vi "INI Input Clusters.vi"() -> (0 "File output directories":T2={"Archive Location"=path "", "Archive Location 2"=path "<Not A Path>", "OutPut Path"=path "", "Directory(s) To Scan Files"=[]}, 1 "FTP CRED Cluster":T4={"Host"="", "UserName"="", "PassWord"="", "FTP File Path"="", "FTP Timeout (S)"=60, "Active or Passive"=FALSE, "ASCII or Binary"=FALSE} {"FTP Timeout (S)" min=0 max=300 step=1}, 2 "Email Notification Cluster":T3, 3 "Email Recipiant List":string[](array[string]), 4 "error out":errorcluster, 5 "time stamp":timestamp, 6 "Site ID":string, 7 "File Management cluster":T1, 8 "Auto FTP":bool, 9 "Auto Archive":bool, 11 "hours old date mod(hours)":u8=2)   [LabVIEW 2011]
uses:
  Controls/FTP Credintials.ctl
  Controls/Ping address and email notify.ctl
  Controls/File Path directories.ctl
  Controls/File Management.ctl
  <vilib>/Utility/sysdir.llb/System Directory Type.ctl
  <vilib>/Utility/config.llb/Read Key (String).vi
  <vilib>/Utility/config.llb/Read Key (Boolean).vi
  <vilib>/Utility/config.llb/Read Key (Path).vi
  <vilib>/Utility/config.llb/Read Key (I32).vi
  <vilib>/Utility/config.llb/Read Key (U32).vi
  <vilib>/Utility/config.llb/NI_LVConfig.lvlib
panel:
  # "File Handling Method"
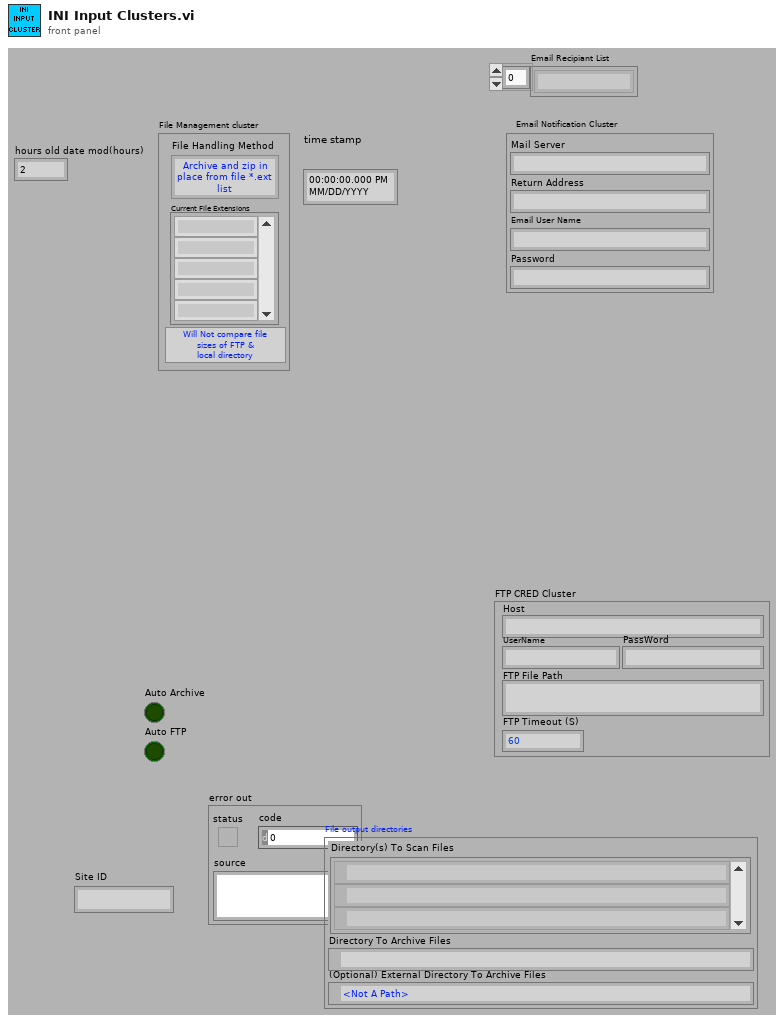
[diagram p1: front panel]
types:
  T1 = typedef "File Management.ctl" = cluster{"Comp File Size":bool, "File Handle Method":enum16{"Archive and zip in place from file *.ext list", "Archive and zip ALL file Types to archive directory", "Archive and zip to archive directory from file *.ext list", "Perform no file management"}, "file extention list":string[]}
  T2 = typedef "File Path directories.ctl" = cluster{"Archive Location":path, "Archive Location 2":path, "OutPut Path":path, "Directory(s) To Scan Files":path[]}
  T3 = typedef "Ping address and email notify.ctl" = cluster{"Mail Server":string, "Return Address":string, "Email User Name":string, "Password":string}
  T4 = typedef "FTP Credintials.ctl" = cluster{"Host":string, "UserName":string, "PassWord":string, "FTP File Path":string, "FTP Timeout (S)":i32, "Active or Passive":bool, "ASCII or Binary":bool}
  T5 = enum16{"Archive and Zip IN Place", "Archive and Zip All File Types", "Archive and Zip from List of File Extensions ", "Perform No File Management"}
  T6 = typedef "System Directory Type.ctl" = i32
  T7 = typedef "NI_LVConfig.lvlib/Config Data RefNum.ctl" = refnum<k1>
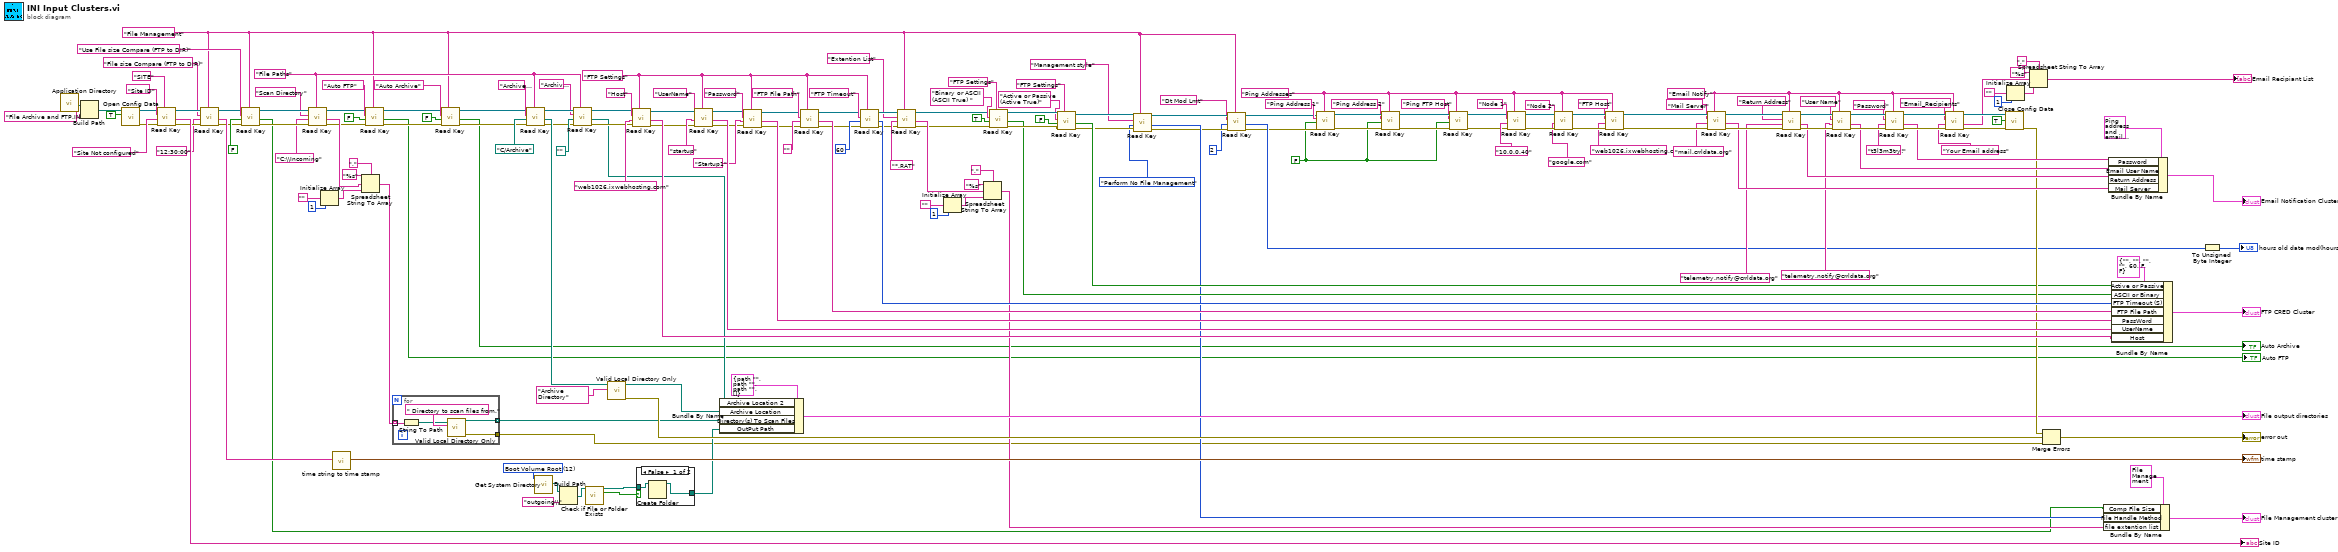
[diagram p0: block diagram]
diagram:
  w1 = FALSE
  w27 = "File Management" ("section")
  w77 = T6 12 items=["User Home"=0, "User Desktop"=1, "User Documents"=2, "User Application Data"=3, "User Preferences"=4, "User Temporary"=5, "Public Documents"=6, "Public Application Data"=7, "Public Preferences"=8, "Public Cache"=13, "System Core Libraries"=9, "System Installed Libraries"=10, "Application Files"=11, "Boot Volume Root"=12] ("system directory type")
  w102 = "FTP Settings" ("name or relative path")
  w91 = "File Paths" ("name or relative path")
  w2 = "Ping Addresses" ("name or relative path")
  w192 = "Email Notify" ("name or relative path")
  n1 = call <vilib>:"Application Directory.vi"() -> ("Application Directory"=w16:path)
  n2 = Build Path(base path=w16, name or relative path="File Archive and FTP.INI") -> (appended path=w140:path)
  n3 = call <vilib>:"Open Config Data.vi"("create file if necessary (T)"=TRUE, "configuration file path"=w140) -> ("error out"=w129:errorcluster, "refnum"=w130:T7)  [unwired: 7 in, 1 out]
  n4 = call-poly <vilib>:"Read Key.vi"("section"="SITE" ("name or relative path"), "error in (no error)"=w129, "default value"="Site Not configured", "key"="Site ID" ("name or relative path"), "refnum"=w130) -> ("error out"=w132:errorcluster, "value"=→"Site ID":string, "refnum out"=w131:T7)  [unwired: 3 in, 1 out]
  n5 = call-poly <vilib>:"Read Key.vi"("section"=w27, "error in (no error)"=w132, "default value"="12:30:00", "key"="File size Compare (FTP to DIR)" ("name or relative path"), "refnum"=w131) -> ("error out"=w120:errorcluster, "value"=w127:string, "refnum out"=w121:T7)  [unwired: 3 in, 1 out]
  n6 = call-poly <vilib>:"Read Key.vi"("section"=w27, "error in (no error)"=w120, "default value"=FALSE ("create file if necessary (T)"), "key"="Use File size Compare (FTP to DIR)" ("name or relative path"), "refnum"=w121) -> ("error out"=w123:errorcluster, "value"=w50:bool, "refnum out"=w122:T7)  [unwired: 3 in, 1 out]
  n7 = call-poly <vilib>:"Read Key.vi"("section"=w91, "error in (no error)"=w123, "default value"="C:\\Incoming", "key"="Scan Directory" ("name or relative path"), "refnum"=w122) -> ("error out"=w23:errorcluster, "value"=w39:string, "refnum out"=w26:T7)  [unwired: 3 in, 1 out]
  n8 = Initialize Array("", 1 ("dimension size")) -> (w40:string[])
  n9 = call "time string to time stamp.vi"("time string example(16:15:00)"=w127) -> ("time stamp"=→"time stamp":timestamp)  [unwired: 10 in]
  n10 = Spreadsheet String To Array(delimiter (Tab)=",", format string="%s", spreadsheet string=w39, array type (2D Dbl)=w40) -> (array=w38:string[])
  n11 = call-poly <vilib>:"Read Key.vi"("section"=w27, "error in (no error)"=w23, "default value"=FALSE, "key"="Auto FTP" ("name or relative path"), "refnum"=w26) -> ("error out"=w22:errorcluster, "value"=→"Auto FTP":bool, "refnum out"=w25:T7)  [unwired: 3 in, 1 out]
  n12 = for {
    tunnel: w38 -> [w199] mode=indexing
    tunnel: [w196] -> w37 mode=indexing
    tunnel: [w195] -> w36
    n13 = String To Path(string=w199) -> (path=w197:path)
    n14 = call "Valid Local Directory Only.vi"("Directory ref"=" Directory to scan files from.", "Path input"=w197) -> ("error out"=w195:errorcluster, "Path output"=w196:path)  [unwired: 8 in]
  }
  n15 = call-poly <vilib>:"Read Key.vi"("section"=w27, "error in (no error)"=w22, "default value"=FALSE, "key"="Auto Archive" ("name or relative path"), "refnum"=w25) -> ("error out"=w21:errorcluster, "value"=→"Auto Archive":bool, "refnum out"=w24:T7)  [unwired: 3 in, 1 out]
  n16 = call-poly <vilib>:"Read Key.vi"("section"=w91, "error in (no error)"=w21, "default value"=path "C:/Archive", "key"="Archive location 1" ("name or relative path"), "refnum"=w24) -> ("error out"=w89:errorcluster, "value"=w138:path, "refnum out"=w88:T7)  [unwired: 3 in, 1 out]
  n17 = call <vilib>:"Get System Directory.vi"("system directory type"=w77) -> ("system directory"=w76:path)  [unwired: 10 in]
  n18 = Build Path(base path=w76, name or relative path="outgoing\\") -> (appended path=w79:path)
  n19 = call-poly <vilib>:"Read Key.vi"("section"=w91, "error in (no error)"=w89, "default value"=path "", "key"="Archive location 2" ("name or relative path"), "refnum"=w88) -> ("error out"=w92:errorcluster, "value"=w85:path, "refnum out"=w97:T7)  [unwired: 3 in, 1 out]
  n20 = call <vilib>:"Check if File or Folder Exists.vi"("path"=w79) -> ("file or folder exists?"=w75:bool, "dup path"=w74:path)  [unwired: 8 in, 1 out]
  n21 = call "Valid Local Directory Only.vi"("Directory ref"="Archive Directory", "Path input"=w138) -> ("error out"=w141:errorcluster, "Path output"=w81:path)  [unwired: 8 in]
  n22 = call-poly <vilib>:"Read Key.vi"("section"=w102, "error in (no error)"=w92, "default value"="web1026.ixwebhosting.com" ("name or relative path"), "key"="Host" ("name or relative path"), "refnum"=w97) -> ("error out"=w93:errorcluster, "value"=w128:string, "refnum out"=w98:T7)  [unwired: 3 in, 1 out]
  n23 = case shown="False" w75 {
    tunnel: w74 -> [w201 w202]
    tunnel: [w200 w202] -> w73
    frame False {
      n24 = Create Folder(path (use dialog)=w201) -> (created path=w200:path)  [unwired: 2 in, 2 out]
    }
    frame True {
    }
  }
  n25 = call-poly <vilib>:"Read Key.vi"("section"=w102, "error in (no error)"=w93, "default value"="startup" ("name or relative path"), "key"="UserName" ("name or relative path"), "refnum"=w98) -> ("error out"=w94:errorcluster, "value"=w117:string, "refnum out"=w99:T7)  [unwired: 3 in, 1 out]
  n26 = Bundle By Name(cluster=T2 {"Archive Location"=path "", "Archive Location 2"=path "", "OutPut Path"=path "", "Directory(s) To Scan Files"=[]} ("File Path Array"), "Archive Location 2"=w85, "Archive Location"=w81, "Directory(s) To Scan Files"=w37, "OutPut Path"=w73) -> (→"File output directories":T2)
  n27 = call-poly <vilib>:"Read Key.vi"("section"=w102, "error in (no error)"=w94, "default value"="Startup1" ("name or relative path"), "key"="Password" ("name or relative path"), "refnum"=w99) -> ("error out"=w95:errorcluster, "value"=w116:string, "refnum out"=w100:T7)  [unwired: 3 in, 1 out]
  n28 = call-poly <vilib>:"Read Key.vi"("section"=w102, "error in (no error)"=w95, "default value"="" ("name or relative path"), "key"="FTP File Path" ("name or relative path"), "refnum"=w100) -> ("error out"=w96:errorcluster, "value"=w115:string, "refnum out"=w101:T7)  [unwired: 3 in, 1 out]
  n29 = call-poly <vilib>:"Read Key.vi"("section"=w102, "error in (no error)"=w96, "default value"=60, "key"="FTP Timeout" ("name or relative path"), "refnum"=w101) -> ("error out"=w63:errorcluster, "value"=w142:i32, "refnum out"=w62:T7)  [unwired: 3 in, 1 out]
  n30 = call-poly <vilib>:"Read Key.vi"("section"=w27, "error in (no error)"=w63, "default value"="*.RAT", "key"="Extention List", "refnum"=w62) -> ("error out"=w61:errorcluster, "value"=w65:string, "refnum out"=w60:T7)  [unwired: 3 in, 1 out]
  n31 = Initialize Array("", 1 ("dimension size")) -> (w70:string[])
  n32 = Spreadsheet String To Array(delimiter (Tab)=",", format string="%s", spreadsheet string=w65, array type (2D Dbl)=w70) -> (array=w56:string[])
  n33 = call-poly <vilib>:"Read Key.vi"("section"="FTP Settings" ("name or relative path"), "error in (no error)"=w61, "default value"=TRUE, "key"="Binary or ASCII (ASCII True) " ("name or relative path"), "refnum"=w60) -> ("error out"=w194:errorcluster, "value"=w72:bool, "refnum out"=w193:T7)  [unwired: 3 in, 1 out]
  n34 = call-poly <vilib>:"Read Key.vi"("section"="FTP Settings" ("name or relative path"), "error in (no error)"=w194, "default value"=FALSE, "key"="Active or Passive (Active True)" ("name or relative path"), "refnum"=w193) -> ("error out"=w54:errorcluster, "value"=w71:bool, "refnum out"=w55:T7)  [unwired: 3 in, 1 out]
  n35 = call-poly <vilib>:"Read Key.vi"("section"=w27, "error in (no error)"=w54, "default value"=T5."Perform No File Management" ("File Handle Method"), "key"="Management style", "refnum"=w55) -> ("error out"=w34:errorcluster, "value"=w52:i32, "refnum out"=w35:T7)  [unwired: 3 in, 1 out]
  n36 = call-poly <vilib>:"Read Key.vi"("section"=w27, "error in (no error)"=w34, "default value"=u32 2, "key"="Dt Mod Lmt" ("name or relative path"), "refnum"=w35) -> ("error out"=w8:errorcluster, "value"=w31:u32, "refnum out"=w12:T7)  [unwired: 3 in, 1 out]
  n37 = call-poly <vilib>:"Read Key.vi"("section"=w2, "error in (no error)"=w8, "default value"=w1, "key"="Ping Address 1" ("Mail Server"), "refnum"=w12) -> ("error out"=w7:errorcluster, "refnum out"=w11:T7)  [unwired: 3 in, 2 out]
  n38 = call-poly <vilib>:"Read Key.vi"("section"=w2, "error in (no error)"=w7, "default value"=w1, "key"="Ping Address 2" ("Mail Server"), "refnum"=w11) -> ("error out"=w6:errorcluster, "refnum out"=w10:T7)  [unwired: 3 in, 2 out]
  n39 = call-poly <vilib>:"Read Key.vi"("section"=w2, "error in (no error)"=w6, "default value"=w1, "key"="Ping FTP Host" ("Mail Server"), "refnum"=w10) -> ("error out"=w5:errorcluster, "refnum out"=w9:T7)  [unwired: 3 in, 2 out]
  n40 = call-poly <vilib>:"Read Key.vi"("section"=w2, "error in (no error)"=w5, "default value"="10.0.0.40", "key"="Node 1" ("Mail Server"), "refnum"=w9) -> ("error out"=w163:errorcluster, "refnum out"=w162:T7)  [unwired: 3 in, 2 out]
  n41 = call-poly <vilib>:"Read Key.vi"("section"=w2, "error in (no error)"=w163, "default value"="google.com", "key"="Node 2" ("Mail Server"), "refnum"=w162) -> ("error out"=w164:errorcluster, "refnum out"=w165:T7)  [unwired: 3 in, 2 out]
  n42 = call-poly <vilib>:"Read Key.vi"("section"=w2, "error in (no error)"=w164, "default value"="web1026.ixwebhosting.com", "key"="FTP Host" ("Mail Server"), "refnum"=w165) -> ("error out"=w167:errorcluster, "refnum out"=w166:T7)  [unwired: 3 in, 2 out]
  n43 = call-poly <vilib>:"Read Key.vi"("section"=w192, "error in (no error)"=w167, "default value"="mail.crrldata.org", "key"="Mail Server" ("Mail Server"), "refnum"=w166) -> ("error out"=w174:errorcluster, "value"=w155:string, "refnum out"=w175:T7)  [unwired: 3 in, 1 out]
  n44 = call-poly <vilib>:"Read Key.vi"("section"=w192, "error in (no error)"=w174, "default value"="telemetry.notify@crrldata.org", "key"="Return Address" ("Return Address"), "refnum"=w175) -> ("error out"=w176:errorcluster, "value"=w154:string, "refnum out"=w179:T7)  [unwired: 3 in, 1 out]
  n45 = call-poly <vilib>:"Read Key.vi"("section"=w192, "error in (no error)"=w176, "default value"="telemetry.notify@crrldata.org", "key"="User Name" ("Email User Name"), "refnum"=w179) -> ("error out"=w177:errorcluster, "value"=w153:string, "refnum out"=w178:T7)  [unwired: 3 in, 1 out]
  n46 = call-poly <vilib>:"Read Key.vi"("section"=w192, "error in (no error)"=w177, "default value"="t3l3m3try!", "key"="Password" ("Password"), "refnum"=w178) -> ("error out"=w188:errorcluster, "value"=w152:string, "refnum out"=w187:T7)  [unwired: 3 in, 1 out]
  n47 = call-poly <vilib>:"Read Key.vi"("section"=w192, "error in (no error)"=w188, "default value"="Your Email address", "key"="Email_Recipients" ("Password"), "refnum"=w187) -> ("error out"=w191:errorcluster, "value"=w189:string, "refnum out"=w190:T7)  [unwired: 3 in, 1 out]
  n48 = call <vilib>:"Close Config Data.vi"("error in (no error)"=w191, "write file if changed (T)"=TRUE, "refnum"=w190) -> ("error out"=w84:errorcluster)  [unwired: 7 in, 1 out]
  n49 = Initialize Array("", 1 ("dimension size")) -> (w180:string[])
  n50 = Spreadsheet String To Array(delimiter (Tab)=",", format string="%s", spreadsheet string=w189, array type (2D Dbl)=w180) -> (array=→"Email Recipiant List":string[])
  n51 = Merge Errors(w84, w141, w36) -> (→"error out":errorcluster)
  n52 = Bundle By Name(cluster=T1 {"Comp File Size"=FALSE, "File Handle Method"=enum."Archive and zip in place from file *.ext list", "file extention list"=[]} ("File Management"), "Comp File Size"=w50, "File Handle Method"=w52, "file extention list"=w56) -> (→"File Management cluster":T1)
  n53 = Bundle By Name(cluster=T3 {"Mail Server"="mail.crrldata.org", "Return Address"="telemetry.notify@crrldata.org", "Email User Name"="telemetry.notify@crrldata.org", "Password"="t3l3m3try!"} ("Email Notification Cluster"), "Password"=w152, "Email User Name"=w153, "Return Address"=w154, "Mail Server"=w155) -> (→"Email Notification Cluster":T3)
  n54 = Bundle By Name(cluster=T4 {"Host"="", "UserName"="", "PassWord"="", "FTP File Path"="", "FTP Timeout (S)"=60, "Active or Passive"=FALSE, "ASCII or Binary"=FALSE} ("FTP Creds"), "Active or Passive"=w71, "ASCII or Binary"=w72, "FTP Timeout (S)"=w142, "FTP File Path"=w115, "PassWord"=w116, "UserName"=w117, "Host"=w128) -> (→"FTP CRED Cluster":T4)
  n55 = To Unsigned Byte Integer(number=w31) -> (unsigned 8bit integer=→"hours old date mod(hours)":u8)
